vi "while_v0_v9.vi"() -> ()   [LabVIEW 2009]
panel:
  in  "Latime impuls":i64(knob)=154 scale=100.0..400.0
  in  "Temporizare intre doua puncte afisate (ms)":dbl(slide)=4.313099041533546 scale=0.0..50.0
  out "Waveform Chart":i64(graph)=92
  in  "stop":bool
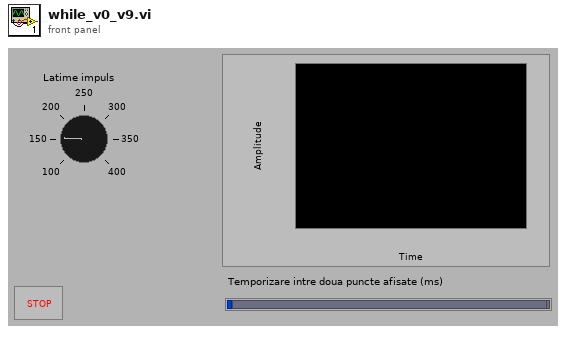
[diagram p1: front panel]
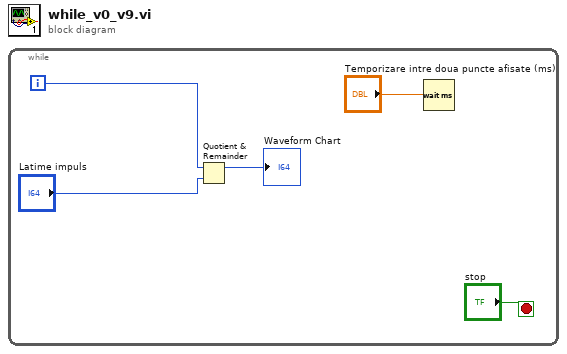
[diagram p0: block diagram]
diagram:
  n1 = while {
    i -> [w2]
    stop <- "stop" stop-if-true
    n2 = Quotient & Remainder(x=w2, y="Latime impuls") -> (x-y*floor(x/y)=→"Waveform Chart":i64)  [unwired: 1 out]
    n3 = Wait (ms)(milliseconds to wait="Temporizare intre doua puncte afisate (ms)") -> ()  [unwired: 1 out]
  }
